vi "Insert Element.vi"(8 "error in (no error)":errorcluster, 9 "Value":bool, 10 "Insert Index":i32, 11 "Boolean_1D in":refnum<class "Boolean_1D.lvclass">) -> (0 "error out":errorcluster, 3 "Boolean_1D out":refnum<class "Boolean_1D.lvclass">)   [LabVIEW 2021, in "Boolean_1D.lvclass"]
uses:
  Boolean_1D.lvclass
  Boolean_1D.lvclass/Boolean_1D.ctl
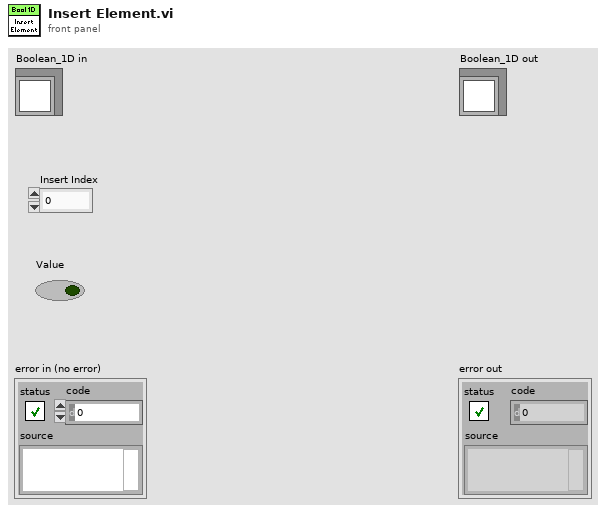
[diagram p1: front panel]
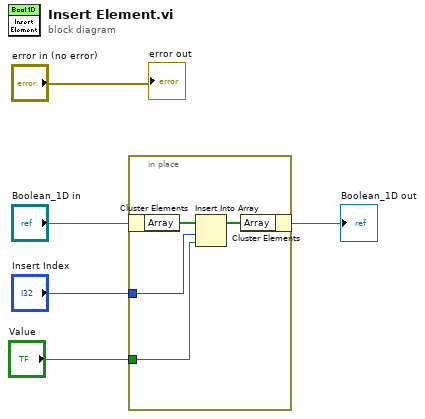
[diagram p0: block diagram]
diagram:
  n1 = in-place {
    in-place-border: "Insert Index" -> [w7]
    in-place-border: "Value" -> [w6]
    n2 = in-place-cluster #1("Boolean_1D in") -> ("Array"=w9:bool[])
    n3 = Insert Into Array(array=w9, index=w7, new element=w6) -> (w8:bool[])
    n4 = in-place-cluster #1("Array"=w8) -> (→"Boolean_1D out":refnum<class "Boolean_1D.lvclass">)
  }
  "error out" <- "error in (no error)"
